vi "Create Table.vi"(7 "Cluster In":variant, 8 "error in (no error)":errorcluster, 10 "Table Name":string, 11 "DatabaseBaseClass In":refnum<class "DatabaseBaseClass.lvclass">) -> (0 "error out":errorcluster, 1 "Column Names":string[](array[string]), 2 "Table Name out":string, 3 "DatabaseBaseClass out":refnum<class "DatabaseBaseClass.lvclass">)   [LabVIEW 2018, in "Database.lvlib" / "DatabaseBaseClass.lvclass"]
uses:
  DatabaseBaseClass.lvclass
  PostgreSQL/PostgreSQL.lvclass
  C:/Projects/SmartGrid/ICDAS/NistPluggableModules/Database/DatabaseBaseClass/DatabaseBaseClass.lvclass
  <vilib>/addons/database/Connection.llb/Conn Execute.vi
  <vilib>/addons/database/Recordset.llb/Rec Destroy - Connection.vi
  <vilib>/addons/database/NI_Database_API.lvlib
  <vilib>/Utility/Data Type/NI_Data Type.lvlib
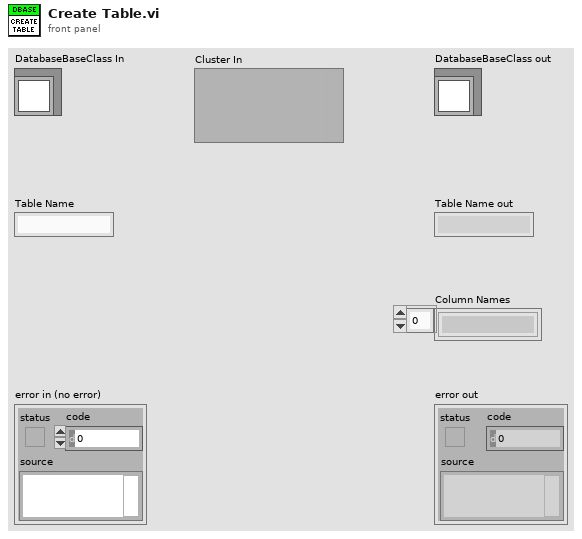
[diagram p1: front panel]
types:
  T1 = typedef "NI_Database_API.lvlib/Conn ObjectReference.ctl" = refnum<k1>
  T2 = typedef "NI_Database_API.lvlib/DB Tools DataTypes.ctl" = enum16{"String", "Long (I32)", "Single (SGL)", "Double (DBL)", "Date/Time", "Binary"}
  T3 = cluster{"name":string, "database data type":T2, "defined size":i32}[]
  T4 = typedef "NI_Data Type.lvlib/Data Type.ctl" = enum8{"Invalid Type", "Void", "I8", "I16", "I32", "I64", "U8", "U16", "U32", "U64", "Single Float", "Double Float", "Extended Float", "Single Complex", "Double Complex", "Extended Complex", "Enum U8", "Enum U16", "Enum U32", "Enum U64", "Single Float With Unit", "Double Float With Unit", "Extended Float With Unit", "Single Complex with Unit", "Double Complex with Unit", "Extended Complex with Unit", "Boolean", "String", "Path", "Picture", "Tag", "Array", "Cluster", "Variant", "LV Variant", "Waveform", "Timestamp", "Digital Waveform", "Digital Data", "ExpressData", "Refnum", "External Data", "VI", "Poly VI", "LabVIEW Class Instance", "Fixed Point"}
  T5 = typedef "NI_Database_API.lvlib/Rec ObjectReference.ctl" = refnum<k1>
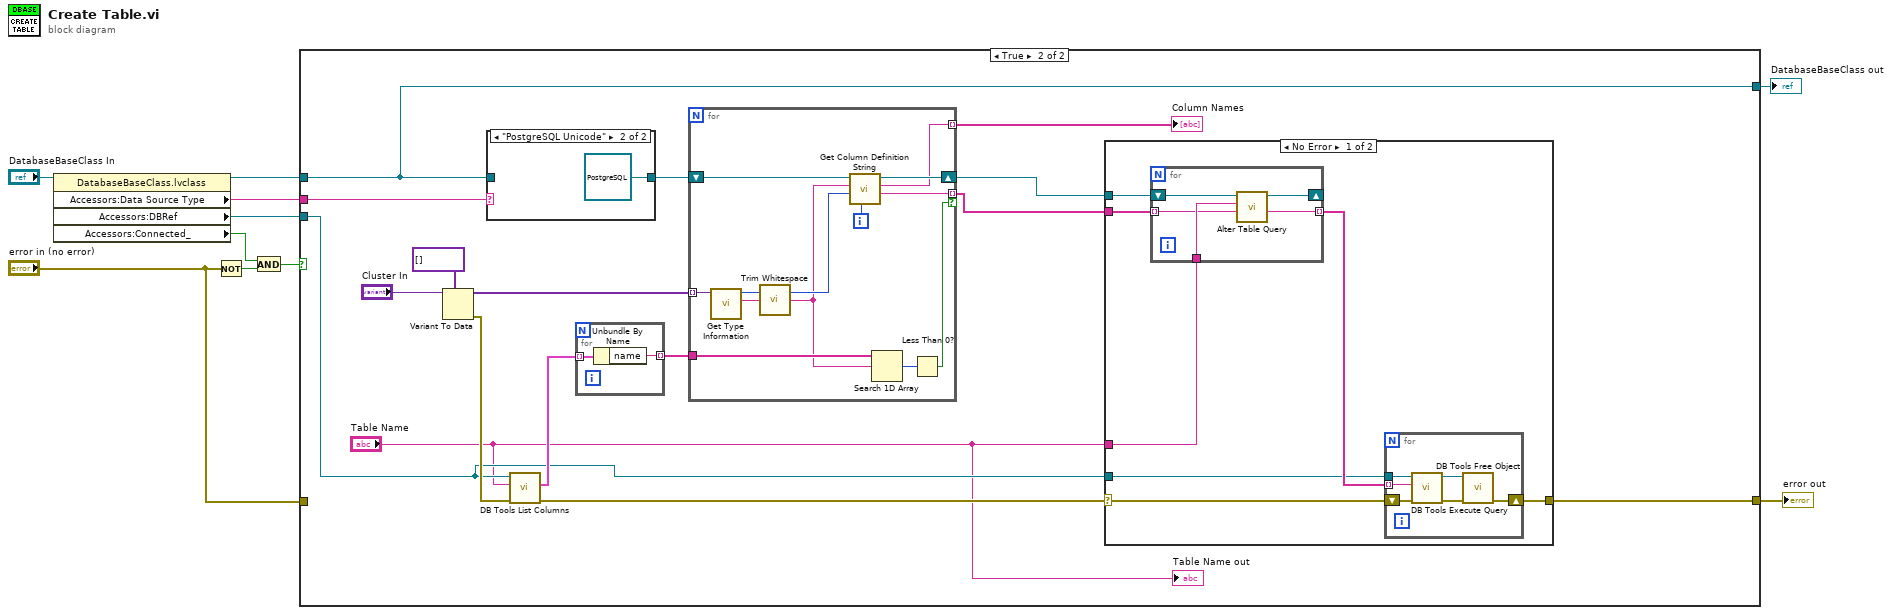
[diagram p0: block diagram]
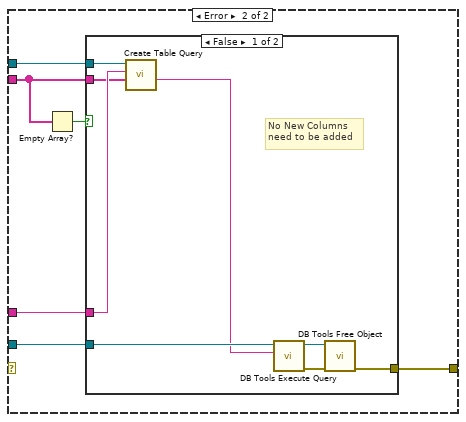
[diagram p3: hidden frame]
diagram:
  n1 = property class="DatabaseBaseClass.lvclass"(reference="DatabaseBaseClass In") -> (reference out=w6:refnum<class "DatabaseBaseClass.lvclass">, "Accessors:Data Source Type"=w1:string, "Accessors:DBRef"=w2:T1, "Accessors:Connected_"=w5:bool)  [unwired: 1 in, 1 out]
  n2 = Not(x="error in (no error)") -> (.not. x?=w7:bool)
  n3 = And(x=w5, y=w7) -> (x .and. y?=w4:bool)
  n4 = case shown="True" w4 {
    tunnel: [w12 w22] -> w10
    tunnel: [w11 w17] -> w8
    tunnel: w6 -> [w11 w17]
    tunnel: "error in (no error)" -> [w12 _]
    tunnel: w2 -> [_ w21]
    tunnel: w1 -> [_ w19]
    frame False {
    }
    frame True {
      n5 = Variant To Data(type=variant[] [] ("appended array"), Variant="Cluster In") -> (data=w13:variant[], error out=w23:errorcluster)  [unwired: 1 in]
      n6 = case shown="\"PostgreSQL Unicode\"" w19 {
        tunnel: [w73 refnum<class "PostgreSQL.lvclass"> refnum ("Database.lvlib:PostgreSQL.lvclass")] -> w18
        tunnel: w17 -> [w73 _]
        frame "False", Default {
        }
        frame "PostgreSQL Unicode" {
        }
      }
      n7 = call <vilib>:"DB Tools List Columns.vi"("error in (no error)"=w23, "table"="Table Name", "connection reference"=w21) -> ("error out"=w28:errorcluster, "column information"=w27:T3)  [unwired: 1 in, 2 out]
      n8 = for {
        tunnel: w27 -> [w76] mode=indexing
        tunnel: [w75] -> w14 mode=indexing
        n9 = Unbundle By Name(w76) -> ("name"=w75:string)
      }
      n10 = for {
        tunnel: w14 -> [w39]
        tunnel: [w31] -> w26 mode=indexing
        tunnel: w13 -> [w37] mode=indexing
        shift-right: [w32] -> w16
        shift-left: w18 -> [w36]
        tunnel: [w30] -> w15 mode=indexing if=w29
        i -> [w33]
        n11 = call <vilib>:"Get Type Information.vi"("Variant"=w37) -> ("Name"=w40:string, "Type"=w35:T4)  [unwired: 6 in, 3 out]
        n12 = call <vilib>:"Trim Whitespace.vi"("string"=w40) -> ("trimmed string"=w34:string)  [unwired: 1 in]
        n13 = call-dynamic "Get Column Definition String.vi"("Column Index (0=Primary Key)"=w33, "Data Type"=w35, "Column Name"=w34, "DatabaseBaseClass in"=w36) -> ("Column Definition String"=w30:string, "Column Name out"=w31:string, "DatabaseBaseClass out"=w32:refnum<class "DatabaseBaseClass.lvclass">)  [unwired: 4 in, 1 out]
        n14 = Search 1D Array(1D array=w39, element=w34) -> (index of element=w38:i32)  [unwired: 1 in]
        n15 = Less Than 0?(x=w38) -> (x < 0?=w29:bool)
      }
      "Column Names" <- w26
      n16 = case shown="No Error" w28 {
        selector: w28 -> [w45 _]
        tunnel: "Table Name" -> [w47 w61]
        tunnel: [w46 w64] -> w22
        tunnel: w21 -> [w43 w63]
        tunnel: w16 -> [w42 w62]
        tunnel: w15 -> [w41 w60]
        frame No Error {
          n17 = for {
            tunnel: w47 -> [w50]
            tunnel: [w48] -> w44 mode=indexing
            shift-right: [w51] -> _
            shift-left: w42 -> [w52]
            tunnel: w41 -> [w49] mode=indexing
            n18 = call-dynamic "Alter Table Query.vi"("Column Definition String"=w49, "Table Name"=w50, "DatabaseBaseClass in"=w52) -> ("Alter Table Query"=w48:string, "DatabaseBaseClass out"=w51:refnum<class "DatabaseBaseClass.lvclass">)  [unwired: 6 in, 1 out]
          }
          n19 = for {
            tunnel: w44 -> [w54] mode=indexing
            shift-right: [w58] -> w46
            shift-left: w45 -> [w53]
            tunnel: w43 -> [w57]
            n20 = call-poly <vilib>:"DB Tools Execute Query.vi"("error in (no error)"=w53, "SQL query"=w54, "connection reference"=w57) -> ("error out"=w56:errorcluster, "recordset reference"=w55:T5)  [unwired: 5 in]
            n21 = call-poly <vilib>:"DB Tools Free Object.vi"("error in (no error)"=w56, "recordset reference"=w55) -> ("error out"=w58:errorcluster)  [unwired: 8 in, 1 out]
          }
        }
        frame Error {
          n22 = Empty Array?(array=w60) -> (empty?=w59:bool)
          n23 = case shown="False" w59 {
            tunnel: [w70 _] -> w64
            tunnel: w63 -> [w69 _]
            tunnel: w62 -> [w68 _]
            tunnel: w61 -> [w67 _]
            tunnel: w60 -> [w65 _]
            frame False {
              # "No New Columns\nneed to be added"
              n24 = call-dynamic "Create Table Query.vi"("Column Definition Strings"=w65, "Table Name"=w67, "DatabaseBaseClass in"=w68) -> ("Create Table Query"=w66:string)  [unwired: 6 in, 2 out]
              n25 = call-poly <vilib>:"DB Tools Execute Query.vi"("SQL query"=w66, "connection reference"=w69) -> ("error out"=w71:errorcluster, "recordset reference"=w72:T5)  [unwired: 6 in]
              n26 = call-poly <vilib>:"DB Tools Free Object.vi"("error in (no error)"=w71, "recordset reference"=w72) -> ("error out"=w70:errorcluster)  [unwired: 8 in, 1 out]
            }
            frame True {
            }
          }
        }
      }
      "Table Name out" <- "Table Name"
    }
  }
  "error out" <- w10
  "DatabaseBaseClass out" <- w8
